vi "Port1 IO (30k) (SubVI).vi"(11 "port 3 hex  string":string="34.5,,,,$56.3,34.556,,,,$67.9") -> (3 "port 3 OK":string)   [LabVIEW 2014]
panel:
  out "size(s)":i32
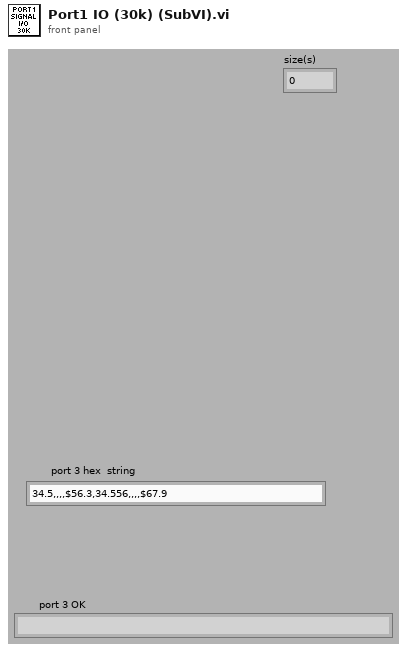
[diagram p1: front panel]
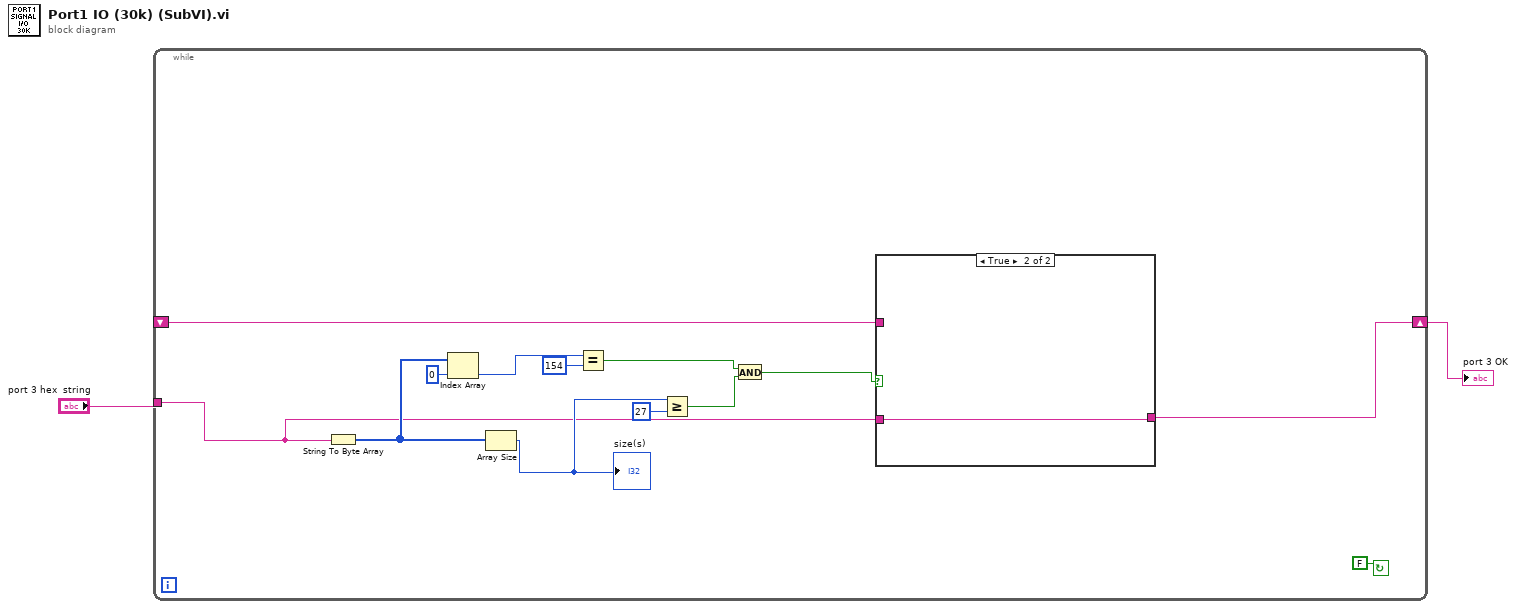
[diagram p0: block diagram]
diagram:
  n1 = while {
    tunnel: "port 3 hex  string" -> [w5]
    shift-right: [w4] -> w1
    shift-left: _ -> [w3]
    stop <- FALSE continue-if-true
    n2 = String To Byte Array(string=w5) -> (unsigned byte array=w14:u8[])
    n3 = Index Array(array=w14, index=0) -> (element=w12:u8)
    n4 = Array Size(array=w14) -> (size(s)=w10:i32)
    "size(s)" <- w10
    n5 = Equal?(x=w12, y=u8 154) -> (x = y?=w7:bool)
    n6 = Greater Or Equal?(x=w10, y=27) -> (x >= y?=w8:bool)
    n7 = And(x=w7, y=w8) -> (x .and. y?=w6:bool)
    n8 = case shown="True" w6 {
      tunnel: w5 -> [_ w17]
      tunnel: [w16 w17] -> w4
      tunnel: w3 -> [w16 _]
      frame False {
      }
      frame True {
      }
    }
  }
  "port 3 OK" <- w1
